vi "Convergence Speed and Computation Time of Adaptive Filters.vi"() -> ()   [LabVIEW 2019]
doc: "This example compares the convergence and computation speeds of the following adaptive filter algorithms: LMS, fast block LMS, and QR-RLS. This VI creates and analyzes one adaptive filter for each algorithm. Each adaptive filter has the same filter length.\n\nAfter you run this VI, notice that the convergence speed of the QR-RLS adaptive filter is the fastest, but the computation speed is the slowest. The convergence speeds of the LMS and fast block LMS adaptive filters are similar, but the computation speed of the fast block LMS adaptive filter is faster than that of the LMS adaptive filter."
uses:
  <vilib>/addons/Adaptive Filters/Create/AFT Create FIR LMS (Real).vi
  <vilib>/addons/Adaptive Filters/Processing/AFT Filter Signal and Update Coefficients (Real, Array).vi
  <vilib>/addons/Adaptive Filters/Create/AFT Create FIR QR-RLS (Real).vi
  <vilib>/addons/Adaptive Filters/NI_AdaptiveFilter.lvlib
panel:
  out "QR-RLS info":string
  out "FBLMS info":string
  out "LMS info":string
  in  "QR-RLS \nForgetting Factor":dbl=0.99 min=0.0 max=1.0 step=0.01
  in  "FBLMS Step Size":dbl=0.001 min=1e-08 step=0.001
  in  "LMS Step Size":dbl=0.001 min=1e-08 step=0.001
  out "Error Signals":dbl[][](graph)
  in  "Filter Length":i32=512 min=2
  out "QR-RLS (ms)":u32
  out "LMS (ms)":dbl
  out "Fast Block LMS (ms)":dbl
  # "Select Help>>Show Context Help and move the cursor over the VI icon of this example for more information."
  # "Computation Time Comparison"
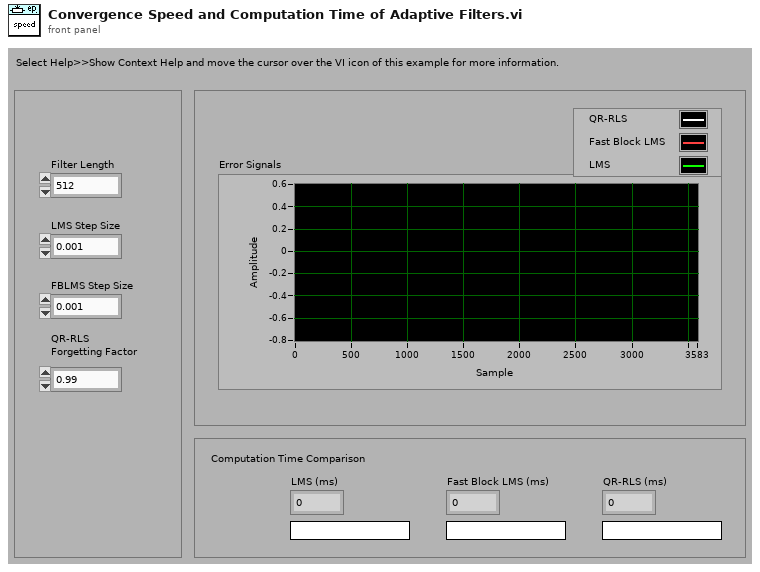
[diagram p1: front panel]
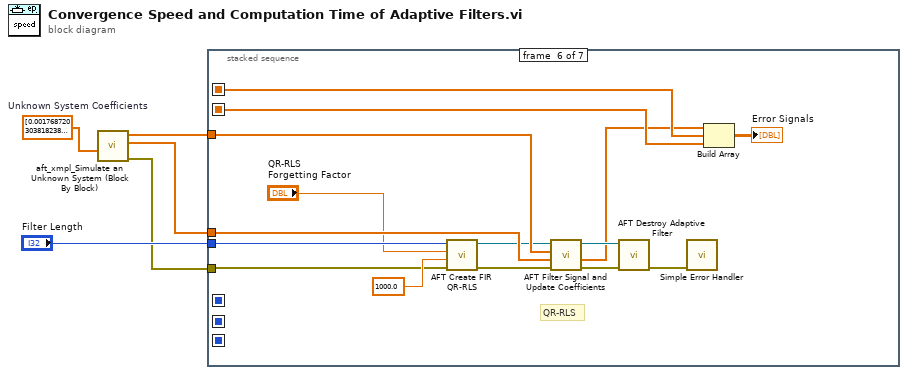
[diagram p0: block diagram]
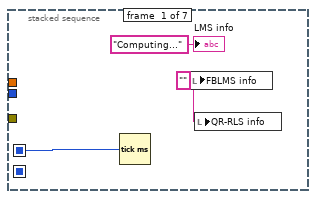
[diagram p2: hidden frame]
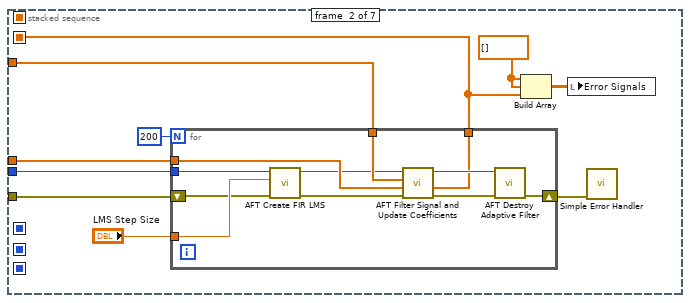
[diagram p3: hidden frame]
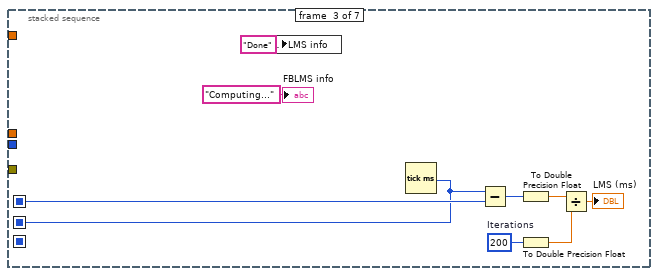
[diagram p4: hidden frame]
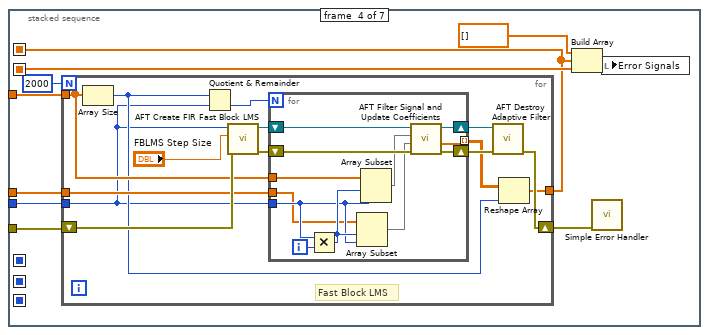
[diagram p5: hidden frame]
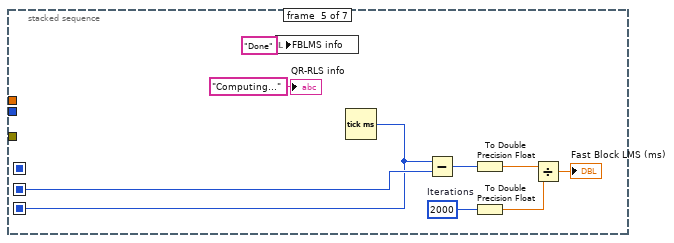
[diagram p6: hidden frame]
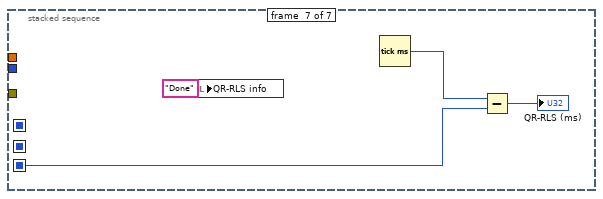
[diagram p7: hidden frame]
diagram:
  w1 = dbl[] [0.0017687203038182385, 0.003309910401378512, -0.001478116721523955, -0.004619432059799202, 0.0019925703728297826, 0.005263544458572513, 0.0024372235607152816, -0.0026069967524432413, 0.005842112100279015, 0.005269794161493996, 0.0031765253411198653, 0.006637344181368461, -0.004722075533337039, -0.011593385544007196, 0.004862664323485264, -0.0014190070162750086, 0.005026007050795865, 0.0035479374138627086, -0.003361611120572154, -0.05, -0.055, -0.04, -0.02, 0.01, 0.02, 0.025, 0.035, 0.047, 0.053, 0.034, 0.011052208374284214, -0.0036582361105590225, 0.002926730612984543, -0.006261394289880111, -0.0033129618153005845, 0.005198195409816674, -0.0007684168484919009, 0.00591801082494993, -0.004946422832583708, 0.008089926926634988, -0.0019701240574926202, 0.0070325566139436205, -0.0034596331706951504, 0.0031419136576151126, -0.003190917762260488, -0.0024559098706700773, 0.00316630812806051, 0.0019936057875049357, 0.0010595890257717063, 0.0014038290612194055, -0.0027659640355617073, -0.0013876548590316088, -0.004992149171985489, 0.01, 0.0010056252280670017, -0.004325332877913205, 0.01, 0.02, -0.0024346180114428926, -0.006781577739216544, 0.003432666982530129, 0.006360797732856513, -0.0009236337042344949, -0.00018971940694013776, -0.0026112611838534972, 0.006992602185473393, 0.004749931445220413, -0.003800811182576462, 0.003944108035041712, -0.004904919925839329, 0.0061893392083196734, -0.0004345633549780014, -0.0015486478558912676, -0.0028791602684276074, 1.4086028525645594e-05, 0.000990042547873076, 0.00011699094801673067, -0.0052366963666595455, -0.002665798497729608, -0.005713641350046967, 0.0018483751751995569, -0.0013345751376356932, 0.00021527964470002353, 0.010184201195733036, 0.0023153567911793674, -0.014222449796367519, 0.009520896904108275, -0.0012595739501401193, 0.004897323831524145, -0.0070440763616523875, -0.0030502637546397, -0.006901230842305007, -0.0038513110689061547, -0.004609190050800657, 0.005706548938394825, 0.0013710607665017747, 3.809836059728197e-05, -0.00591219375224786, 0.005804809641793159, 0.004764632040202399, 0.0076695988294999545, 0.01, 0.03, 0.05, 0.04, 0.02, -0.0127271289746406, -0.01516194267856794, 0.0028110128605449212, 0.0011738641111162151, -0.0012857994895649288, 0.004263543289976114, -0.003674869314334217, 0.009556015543482402, 0.002489832594054652, -0.005996418179406442, 0.006331218227312546, -0.0064207853482578315, 0.003311862154237889, -0.000955288977224918, 0.0012562208127762015, -0.0023691173826360843, -0.014438040379192016, -0.002214388776364357, 0.008395823224282738, 0.00826412699407891, 0.0012646272838441731, -0.002165263590393799, 0.0002940205937293824, 0.00046177431511072644, -0.001920026430992717, 0.0006121760545153992, 0.0006225481643720151, 0.00026201207562547897, -0.006778520738264402, -0.001256554165000527, 0.008809157516655616, 0.0025607655026032424, -0.0009489918703505415, 8.239364931448987e-05, 0.0019955437250800414, 0.0008386602446357169, 0.012703393574022474, 0.00355922287129002, -0.0007851316888136418, 0.00959348942578702, 0.009530982268201003, -0.004853489344748983, 0.0016031838881485686, -0.010519647173388552, 0.008860178829855896, 0.0001510099869714823, 0.03, -0.01, -0.015, -0.035, -0.00013320604368074646, 0.004007870773181195, -0.0043589271965922645, 0.005561053344576156, -0.0004941879907364923, -0.0013244488412728834, -0.0017482680888189562, 0.0029960604613339663, 0.0031814496833029765, 0.007259699839898215, -0.0040720188008857095, -0.004483037340217165, 0.0013475522940216867, 0.0019969456362042485, -0.0011545138717414215, 0.0038200347611301697, 0.004471407945791518, 3.6228502175092e-05, -0.006690685698674373, -0.0002015653415380347, -0.000770587924412587, -0.0010887589932588966, 0.0010425505500961032, 0.0015857753879059, 0.02, 0.032, 0.012, 0.0033525120298580737, -0.0044016129264833875, 0.002709468590239712, 0.0025776908997332776, 0.00028250172997961, 0.005127577790311253, 0.003573125010679203, -0.004271454173669076, 0.006322694759883522, -0.006052284959693702, -0.0024643146233968493, -9.095570963796674e-05, 0.001996464371178897, 0.00046518565440334424, 0.0019679329979912096, -0.003702071527553143, 0.003524586942818637, 0.006936369645745196, 0.0013812554032625066, -0.005259920326912177, 0.01075111469067106, -0.009899012646386762, 0.002681940912629616, 0.0026668001135738886, -0.00415144373482893, -0.003984850412229487, 0.005126659425844433, 0.004437301714107484, 0.004096337116260746, 0.007858491462627968, -0.0027900179995245804, 0.004253193414256363, -0.00338862346012873, -0.006795552635912255, -0.00358413698580997, -0.0026858057946579075, -0.0008731078879112253, -0.000349057291337621, -0.006225357165172573, 0.0068062127573739716, -0.003740667415656732, -0.004745853741234565, 0.004843395288340839, 0.00990096261848414, 0.0010364677807490747, -0.005555953629618369, -0.010532718356965882, 0.005195012426740025, -0.00625353037310407, -0.00499223201963367, 0.0032842532491144058, 0.011111507249167816, -0.004558283207160444, -0.0009493453639189572, 0.004330689208295522, 0.0011632130727379617, -0.002074335648599739, 0.000943554774206769, 0.0008376233888650976, -0.0033424492109705144, 0.009615250746216523, 0.007887659246972059, 0.006282589869639402, -0.001101754418762132, 0.00732314604308056, -0.0027003305899687214, -0.004340553046981131, 0.0011551116308410449, 0.005465357484435472, 0.005373730333319386, 0.001589426324243375, 0.002884347605524919, -0.005583831699664686, -0.0019958112865996985, -0.0048327734573494555, 0.003121046841227656, 0.011603844499711413, 0.001403690344139859, 0.0013935828042601045, 0.004781110796897716, 0.003254949888398519, 0.009066331843973374, -0.002647534945073365, 0.004357633222107237, -0.005698889588347418, -0.004838162045632235, 0.0010461168423915924, -0.002334618300635773, 0.005504545842227033, -0.006448484935966947, 0.002653858669567252, -0.003069021890032611, 0.0014443889179892727, 0.005924226714331932, -0.009546532275929756, 0.0013194638871403847, 0.0006014993481320031, -0.006784525874344193, -0.006296764058398797, -0.0020148149409728662, -0.01757709947322435, -0.003403770598702304, -0.002764742170669352, 0.0017448721093241836, -0.0028496552331979956, -0.005967230867858146, 0.0013593193466581571, -0.004554179589625983, -0.0005395458990457037, 0.004698919858085422, -0.007833375970934798, 0.004148449797227988, -0.001006283265156829, 0.006762013894188109, -0.0003145841514429291, -0.0014421975271376609, 0.002730744174736778, -0.004514507938754639, -0.0012142460446779174, -0.0014263529879642808, 0.012, 0.02, -0.007597717587842824, 0.0037697891973044228, -0.01, -0.013, -0.010412344667943458, -0.004393430182915761, -0.002740627513586221, 0.00222041628463806, -0.00015873555347002176, -0.007099803253715512, 0.002010534208396422, -0.0028110145062755225, -0.0007262053667323782, -0.0024958939919888824, -0.0008067763058028488, -0.007042978447707788, -0.0035681748290683412, 0.000729405788252263, -0.0001688759649006347, 0.0017607857950298726, -0.0019421135288569815, -0.0026899195217946503, 0.004126099679062706, -0.006654429646841175, -9.148565563200602e-05, -0.0020552399098966857, 0.00648481370956031, 0.0021420831665986966, -0.0020420956451124507, -0.0032083873202158305, 0.0011877412512870094, -0.009917456320430278, -0.0036222764319343076, -0.00266373168395064, 0.0019568451956730247, 0.0009340921962064619, 0.004667650312274363, -0.00393348047444334, 0.0023144779414032337, 0.002191023452212552, 8.699492361259907e-05, 6.22929932814311e-05, -0.0006414588117240494, -0.000246286737969977, -0.008399156457753838, -0.004042537089553992, 0.003237744207928505, -0.0004758023138765523, 0.004354376000956885, -0.0046855964701936915, -0.000674869483064684, -0.010109941628028267, -0.0019183313203903947, -0.0037082683163142155, 0.005635843455217586, -0.0031726570253010657, 0.002569808736812313, 0.01012255478320051, 0.0013667805173206596, -0.007443021879934841, 0.0007086780950365098, -4.230932439487779e-05, 0.00011384532040662788, 1.806934454506236e-05, 0.0027869839946655715, 0.006862365882408016, -0.00285986173749602, 0.0033074181275176847, 0.0014230939822999884, -0.0016513319885660962, -0.0061490572606759395, 0.0002960975656633335, -0.002169992448222367, -0.007498098114608933, -9.52143176890296e-05, -0.00420465126534504, -0.005891459584701565, -0.005595594734426555, -0.004039576878697208, -0.0012620388475528975, -0.001337401195787844, 0.0031891574600993577, -0.006931577177447051, 0.002968919568786009, 0.009581524842130942, -0.002413534663740632, -0.0032886682198828084, 1.6501661866380983e-06, 0.002407149166499771, -0.0040932545649498605, 0.0003976069887019553, -0.008344774365618342, 0.0010907994823554973, 0.006408275603950336, -0.002172053877951578, 0.0030031265226455445, -0.01, -0.025, -0.006896368357649993, 0.0014453324214440963, -0.00027650227463950344, 0.016246, 0.005240157152894915, 0.006550405469729321, 0.008050920332667447, -0.010033307565564236, -0.008957707334461346, 0.002900158637661118, -0.00538581848771917, -0.0007997603744071992, -0.004464552728430399, 0.006642687637635623, 0.0012383568032714404, 0.004417376522172382, -0.00865444372799693, -0.0008432848420495423, -0.0003959612495558097, 0.005914973783884217, 0.00296424058142418, 0.002040601650139498, -0.0024135129750677917, -0.0018108899619926192, -0.0003917426807699802, 0.008370768085628227, 0.006839124729325788, -0.005169044017416361, 0.004095933293549, -0.007635021721114593, 0.003497056458290858, 0.004837217809455041, -0.00012665304702670524, 0.0014419959233279186, -0.0033583382925281013, -0.009207305281479181, -0.007522432499569415, 0.0071019078305083255, 0.004097440093152365, 0.004287532536653536, -1.1962621121723216e-05, 0.00031712906201941486, 0.00046900056938096546, 0.0029999589246177245, 0.005707862677563847, 0.009793391706896649, -0.0019564394415165776, -0.0038190132308775224, -0.002485259536803924, -0.00013066138142336703, -0.0006518373512934251, 0.010009614902164623, 0.0036855901173668943, -0.004253805905738769, 0.005843744798962357, -0.008909205404961961, -0.0008090850464462802, 0.0026479238342882573, 0.012254803350318755, -0.007747657427436024, -0.009095675410509802, -0.0021364137535619366, 0.011766327215445049, -0.003834430633187085, 0.00035986036508913654, -0.0046659637394370675, 0.0026388037900242386, 0.0036436455380764415, -0.002445926710026739, -0.00014294989687897608, -0.0024908886503159314, -0.00660285441911065, -8.980399078747211e-07, 0.00027803931211150374, 0.001902086091396913, -0.005197811166509313, 0.008541303938008334, -0.010924925080668462, 0.005775550945475447, -0.005033578686136635, 0.0017180580693640793, -0.00532182222957612, -0.0031096541043942796, -0.003383321732726488, -0.004555388725432587, -0.006593658561601619, 0.00580571451934701, 0.0028384150603862467, -0.003257527653178708, 0.010652027301902928, 0.004875971890010786, 0.00921860280618525, -0.009168313082167241, 0.0006048895827707551, 0.00396852782834772, -0.0017959481502440226, -0.0003070846070871938, -0.007315550910261663, -0.00279018088609701, -0.00369834373597139, -0.000849166649009762, 0.0036354433402297093, -0.0037585459253197794, 0.0056801374693337256, -0.0008835456203011095, -0.006676518117936941, 0.004207345300034022, 0.0008639190122816241, -0.004590227220307338]  # Unknown System Coefficients
  n1 = call "aft_xmpl_Simulate an Unknown System (Block By Block).vi"("unknown system coefficients"=w1) -> ("error out"=w2:errorcluster, "response signal"=w5:dbl[], "stimulus signal"=w3:dbl[])  [unwired: 3 in, 5 out]
  n2 = stacked-sequence {
    seq-local: [_ w14 _ _ _ _ _] -> [_ _ _ w45 _ w87 _]
    seq-local: [_ _ _ w43 _ _ _] -> [_ _ _ _ _ w88 _]
    seq-local: [w8 _ _ _ _ _ _] -> [_ _ w36 _ _ _ _]
    seq-local: [_ _ w35 _ _ _ _] -> [_ _ _ _ w81 _ _]
    seq-local: [_ _ _ _ w79 _ _] -> [_ _ _ _ _ _ w100]
    tunnel: w3 -> [_ w18 _ w47 _ w96 _]
    tunnel: w5 -> [_ w17 _ w48 _ w95 _]
    tunnel: "Filter Length" -> [_ w16 _ w46 _ w94 _]
    tunnel: w2 -> [_ w10 _ w40 _ w84 _]
    frame #0 {
      w6 = "" ("FBLMS info")
      n3 = Tick Count (ms)() -> (millisecond timer value=w8:u32)
      n4 = local write "FBLMS info"(w6) -> ()
      n5 = local write "QR-RLS info"(w6) -> ()
      "LMS info" <- "Computing..." ("LMS info")
    }
    frame #1 {
      w12 = dbl[] [] ("element")
      n6 = for {
        N: 200 -> [_]
        tunnel: w18 -> [w27]
        tunnel: w17 -> [w26]
        tunnel: w16 -> [w25]
        tunnel: "LMS Step Size" -> [w24]
        tunnel: [w21] -> w14
        shift-right: [w19] -> w9
        shift-left: w10 -> [w20]
        n7 = call-poly <vilib>:"AFT Create FIR LMS.vi"("error in (no error)"=w20, "step size"=w24, "filter length"=w25) -> ("error out"=w22:errorcluster, "adaptive filter out"=w23:refnum<k20>)  [unwired: 1 in, 6 out]
        n8 = call-poly <vilib>:"AFT Filter Signal and Update Coefficients.vi"("error in (no error)"=w22, "d(n)"=w26, "x(n)"=w27, "adaptive filter in"=w23) -> ("error out"=w29:errorcluster, "e(n)"=w21:dbl[], "adaptive filter out"=w28:refnum<k20>)  [unwired: 2 in, 3 out]
        n9 = call <vilib>:"AFT Destroy Adaptive Filter.vi"("error in (no error)"=w29, "adaptive filter in"=w28) -> ("error out"=w19:errorcluster)  [unwired: 9 out]
      }
      n10 = Build Array(w12, w12, w14) -> (w13:dbl[][])
      n11 = local write "Error Signals"(w13) -> ()
      n12 = call <vilib>:"Simple Error Handler.vi"("error in (no error)"=w9) -> ()  [unwired: 1 in, 8 out]
    }
    frame #2 {
      w32 = u32 200  # Iterations
      n13 = local write "LMS info"("Done" ("LMS info")) -> ()
      n14 = Tick Count (ms)() -> (millisecond timer value=w35:u32)
      n15 = Subtract(x=w35, y=w36) -> (x-y=w34:u32)
      n16 = To Double Precision Float(number=w34) -> (double precision float=w31:dbl)
      n17 = To Double Precision Float(number=w32) -> (double precision float=w30:dbl)
      n18 = Divide(x=w31, y=w30) -> (x/y=→"LMS (ms)":dbl)
      "FBLMS info" <- "Computing..." ("FBLMS info")
    }
    frame #3 {
      n19 = for {
        N: 2000 -> [_]
        tunnel: w48 -> [w58]
        tunnel: w47 -> [w56]
        tunnel: w46 -> [w53]
        tunnel: [w49] -> w43
        shift-right: [w62] -> w39
        shift-left: w40 -> [w61]
        # "Fast Block LMS"
        n20 = Array Size(array=w56) -> (size(s)=w54:i32)
        n21 = Quotient & Remainder(x=w54, y=w53) -> (floor(x/y)=w55:i32)  [unwired: 1 out]
        n22 = call <vilib>:"AFT Create FIR Fast Block LMS.vi"("error in (no error)"=w61, "step size"="FBLMS Step Size", "filter length"=w53) -> ("error out"=w50:errorcluster, "adaptive filter out"=w51:refnum<k20>)  [unwired: 1 in, 6 out]
        n23 = for {
          N: w55 -> [_]
          tunnel: [w70] -> w57 mode=indexing
          shift-right: [w73] -> w59
          shift-left: w50 -> [w72]
          tunnel: w53 -> [w67]
          tunnel: w58 -> [w63]
          tunnel: w56 -> [w65]
          shift-right: [w74] -> w60
          shift-left: w51 -> [w68]
          i -> [w71]
          n24 = Multiply(x=w67, y=w71) -> (x*y=w69:i32)
          n25 = Array Subset(array=w63, index=w69, length=w67) -> (w66:dbl[])
          n26 = Array Subset(array=w65, index=w69, length=w67) -> (w64:dbl[])
          n27 = call-poly <vilib>:"AFT Filter Signal and Update Coefficients.vi"("error in (no error)"=w72, "d(n)"=w66, "x(n)"=w64, "adaptive filter in"=w68) -> ("error out"=w73:errorcluster, "e(n)"=w70:dbl[], "adaptive filter out"=w74:refnum<k20>)  [unwired: 2 in, 3 out]
        }
        n28 = call <vilib>:"AFT Destroy Adaptive Filter.vi"("error in (no error)"=w59, "adaptive filter in"=w60) -> ("error out"=w62:errorcluster)  [unwired: 9 out]
        n29 = Reshape Array(w57, w54) -> (w49:dbl[])
      }
      n30 = Build Array(dbl[] [] ("element"), w43, w45) -> (w44:dbl[][])
      n31 = call <vilib>:"Simple Error Handler.vi"("error in (no error)"=w39) -> ()  [unwired: 1 in, 8 out]
      n32 = local write "Error Signals"(w44) -> ()
    }
    frame #4 {
      w77 = u32 2000  # Iterations
      n33 = local write "FBLMS info"("Done" ("FBLMS info")) -> ()
      n34 = Tick Count (ms)() -> (millisecond timer value=w79:u32)
      n35 = Subtract(x=w79, y=w81) -> (x-y=w80:u32)
      n36 = To Double Precision Float(number=w80) -> (double precision float=w76:dbl)
      n37 = To Double Precision Float(number=w77) -> (double precision float=w75:dbl)
      n38 = Divide(x=w76, y=w75) -> (x/y=→"Fast Block LMS (ms)":dbl)
      "QR-RLS info" <- "Computing..." ("QR-RLS info")
    }
    frame #5 {
      # "QR-RLS"
      n39 = call-poly <vilib>:"AFT Create FIR QR-RLS.vi"("error in (no error)"=w84, "regularization factor"=1000.0 ("regulation parameter"), "forgetting factor"="QR-RLS \nForgetting Factor", "filter length"=w94) -> ("error out"=w91:errorcluster, "adaptive filter out"=w90:refnum<k20>)  [unwired: 6 out]
      n40 = call-poly <vilib>:"AFT Filter Signal and Update Coefficients.vi"("error in (no error)"=w91, "d(n)"=w95, "x(n)"=w96, "adaptive filter in"=w90) -> ("error out"=w98:errorcluster, "e(n)"=w86:dbl[], "adaptive filter out"=w97:refnum<k20>)  [unwired: 2 in, 3 out]
      n41 = call <vilib>:"AFT Destroy Adaptive Filter.vi"("error in (no error)"=w98, "adaptive filter in"=w97) -> ("error out"=w85:errorcluster)  [unwired: 9 out]
      n42 = call <vilib>:"Simple Error Handler.vi"("error in (no error)"=w85) -> ()  [unwired: 1 in, 8 out]
      n43 = Build Array(w86, w88, w87) -> (→"Error Signals":dbl[][])
    }
    frame #6 {
      n44 = local write "QR-RLS info"("Done" ("QR-RLS info")) -> ()
      n45 = Tick Count (ms)() -> (millisecond timer value=w101:u32)
      n46 = Subtract(x=w101, y=w100) -> (x-y=→"QR-RLS (ms)":u32)
    }
  }
